vi "Temperatura.vi"() -> (0 "Œrednia temperatura":dbl, 1 "Wartoœæ ciœnienia atmosferycznego":dbl)   [LabVIEW 2024]
uses:
  <vilib>/httpClient/LabVIEWHTTPClient.lvlib
panel:
  out "API w JSON":string
  in  "URL":string="https://weather.visualcrossing.com/VisualCrossingWebServices/rest/services/timeline/Lublin%2CPoland?unitGroup=metric&key=LGSF7VCA2FM6L7WC6KLKWNN58&contentType=json"
  # ". . ."
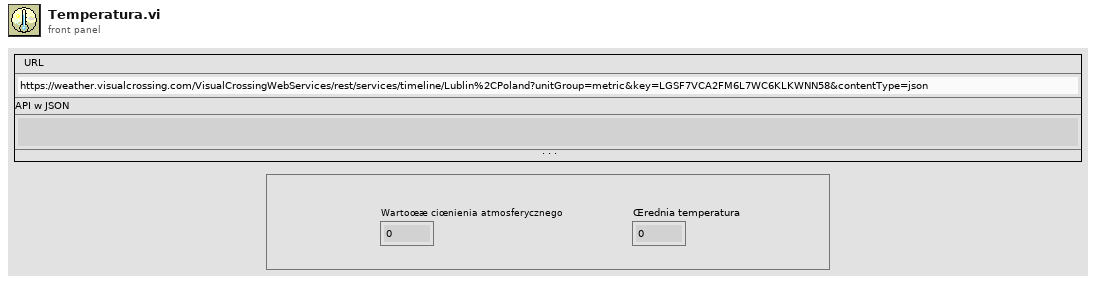
[diagram p1: front panel]
types:
  T1 = typedef "LabVIEWHTTPClient.lvlib/ClientHandle.ctl" = refnum<k1>
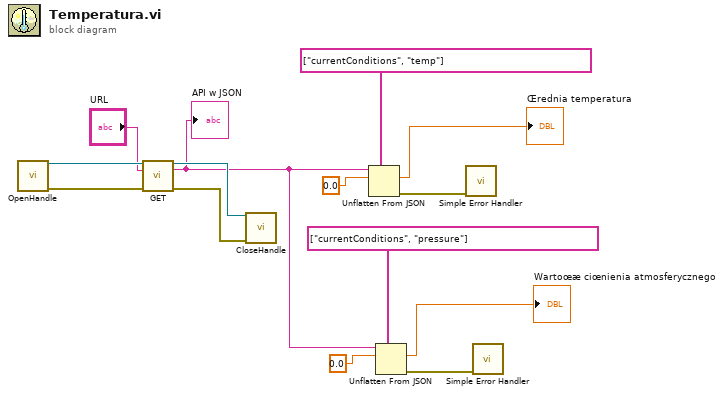
[diagram p0: block diagram]
diagram:
  n1 = call <vilib>:"OpenHandle.vi"() -> ("client handle out"=w14:T1, "error out"=w13:errorcluster)  [unwired: 14 in]
  n2 = call <vilib>:"GET.vi"("client handle"=w14, "url"="URL", "error in (no error)"=w13) -> ("client handle out"=w10:T1, "body"=w1:string, "error out"=w11:errorcluster)  [unwired: 9 in, 1 out]
  "API w JSON" <- w1
  n3 = call <vilib>:"CloseHandle.vi"("client handle"=w10, "error in (no error)"=w11) -> ()  [unwired: 13 in, 1 out]
  n4 = Unflatten From JSON(path=string[] ["currentConditions", "temp"], JSON string=w1, type and defaults=0.0) -> (value=→"Œrednia temperatura":dbl, error out=w9:errorcluster)  [unwired: 4 in]
  n5 = Unflatten From JSON(path=string[] ["currentConditions", "pressure"], JSON string=w1, type and defaults=0.0) -> (value=→"Wartoœæ ciœnienia atmosferycznego":dbl, error out=w5:errorcluster)  [unwired: 4 in]
  n6 = call <vilib>:"Simple Error Handler.vi"("error in (no error)"=w9) -> ()  [unwired: 4 in, 5 out]
  n7 = call <vilib>:"Simple Error Handler.vi"("error in (no error)"=w5) -> ()  [unwired: 4 in, 5 out]
